vi "GetCoincidenceRatio.vi"(1 "lateral peaks":u32=2 min=2 max=10 step=2, 2 "center peak (µs)":dbl format="%.2f", 3 "histogram":u32[](array[numeric])) -> (0 "coincidence ratio":dbl format="%.2f")   [LabVIEW 2009]
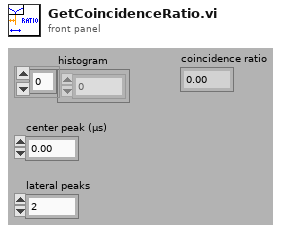
[diagram p1: front panel]
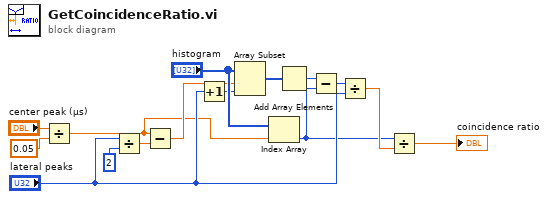
[diagram p0: block diagram]
diagram:
  n1 = Divide(x="center peak (µs)", y=0.05) -> (x/y=w1:dbl)
  n2 = Divide(x="lateral peaks", y=u32 2) -> (x/y=w7:dbl)
  n3 = Subtract(x=w1, y=w7) -> (x-y=w2:dbl)
  n4 = Increment(x="lateral peaks") -> (x+1=w3:u32)
  n5 = Array Subset(array="histogram", index=w2, length=w3) -> (w8:u32[])
  n6 = Index Array(array="histogram", index=w1) -> (element=w11:u32)
  n7 = Add Array Elements(numeric array=w8) -> (sum=w10:u32)
  n8 = Subtract(x=w10, y=w11) -> (x-y=w13:u32)
  n9 = Divide(x=w13, y="lateral peaks") -> (x/y=w15:dbl)
  n10 = Divide(x=w11, y=w15) -> (x/y=→"coincidence ratio":dbl)
